vi "Notifier to Command String.vi"(11 "NotifierReff":T1) -> (3 "String":string)   [LabVIEW 2013]
doc: "Takes the MB sail and rudder commands (-1 to 1 for rudder, 0 to 1 for sails) and translates that into a command string for the arbotix board.\n\nEric Schneider, April 2014"
uses:
  Data/TypeDefs/Notifiers.ctl
  Data/TypeDefs/UTM Location.ctl
  Data/TypeDefs/Sail Set Suggestions.ctl
  Data/TypeDefs/Rudder Set Suggestions.ctl
  Data/TypeDefs/OverrideInformation.ctl
  Data/TypeDefs/OverrideMode.ctl
  Data/TypeDefs/MotorSetup.ctl
  Data/TypeDefs/DynamixelSetupInfo.ctl
  Data/TypeDefs/AirmarStatus.ctl
  Data/TypeDefs/HardwareOnline.ctl
  Data/TypeDefs/DynamixelCycleTracker.ctl
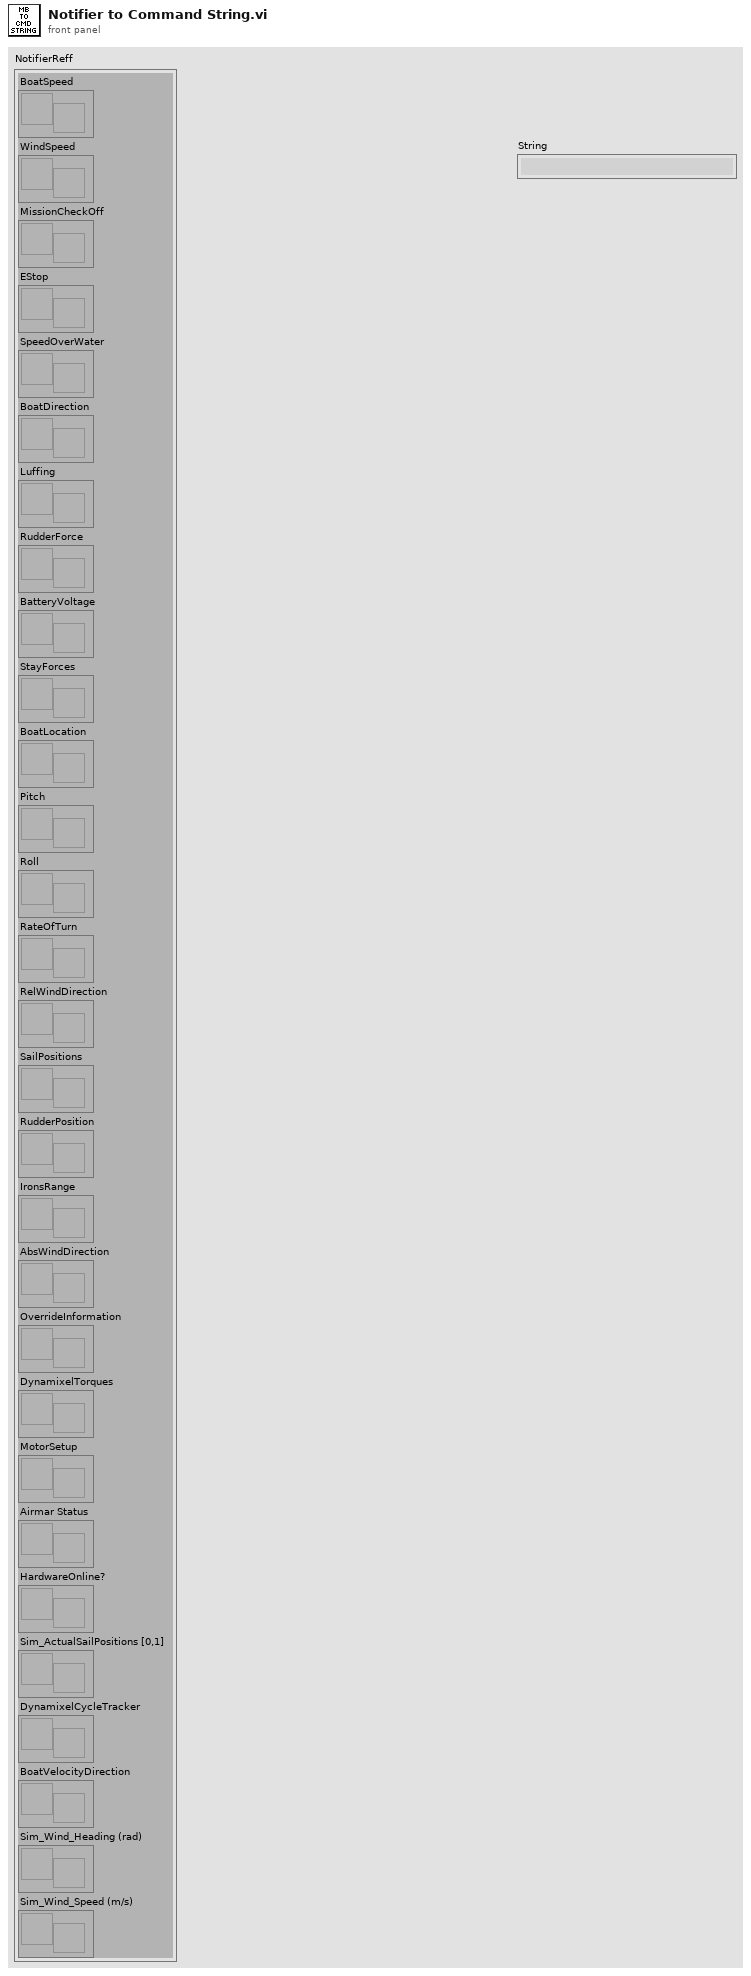
[diagram p1: front panel]
types:
  T1 = typedef "Notifiers.ctl" = cluster{"BoatSpeed":refnum<notifier>, "WindSpeed":refnum<notifier>, "MissionCheckOff":refnum<notifier>, "EStop":refnum<notifier>, "SpeedOverWater":refnum<notifier>, "BoatDirection":refnum<notifier>, "Luffing":refnum<notifier>, "RudderForce":refnum<notifier>, "BatteryVoltage":refnum<notifier>, "StayForces":refnum<notifier>, "BoatLocation":refnum<notifier>, "Pitch":refnum<notifier>, "Roll":refnum<notifier>, "RateOfTurn":refnum<notifier>, "RelWindDirection":refnum<notifier>, "SailPositions":refnum<notifier>, "RudderPosition":refnum<notifier>, "IronsRange":refnum<notifier>, "AbsWindDirection":refnum<notifier>, "OverrideInformation":refnum<notifier>, "DynamixelTorques":refnum<notifier>, "MotorSetup":refnum<notifier>, "Airmar Status":refnum<notifier>, "HardwareOnline?":refnum<notifier>, "Sim_ActualSailPositions [0,1]":refnum<notifier>, "DynamixelCycleTracker":refnum<notifier>, "BoatVelocityDirection":refnum<notifier>, "Sim_Wind_Heading (rad)":refnum<notifier>, "Sim_Wind_Speed (m/s)":refnum<notifier>}
  T2 = typedef "OverrideInformation.ctl" = cluster{"OverrideMode":T3, "SailSetting":T4, "Rudder Setpoint":T5}
  T3 = typedef "OverrideMode.ctl" = enum16{"None", "Rudder", "Sails", "Both"}
  T4 = typedef "Sail Set Suggestions.ctl" = cluster{"MainSailSuggestion":dbl, "JibSailSuggestion":dbl}
  T5 = typedef "Rudder Set Suggestions.ctl" = dbl
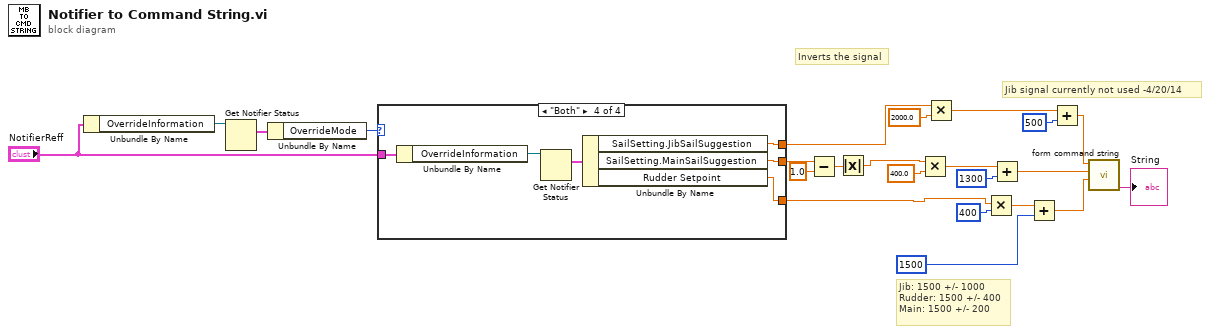
[diagram p0: block diagram]
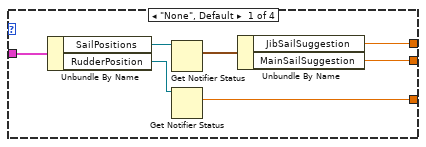
[diagram p2: hidden frame]
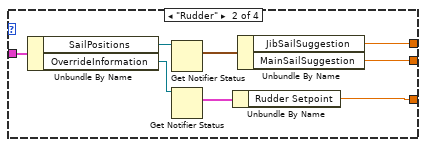
[diagram p3: hidden frame]
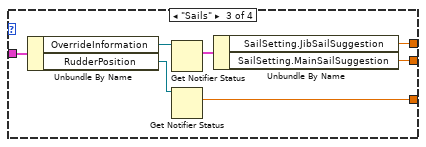
[diagram p4: hidden frame]
diagram:
  # "Jib signal currently not used -4/20/14"
  # "Inverts the signal"
  # "Jib: 1500 +/- 1000\nRudder: 1500 +/- 400\nMain: 1500 +/- 200"
  n1 = Unbundle By Name("NotifierReff") -> ("OverrideInformation"=w8:refnum<notifier>)
  n2 = Get Notifier Status(notifier=w8) -> (current notification=w7:T2)  [unwired: 1 in, 4 out]
  n3 = Unbundle By Name(w7) -> ("OverrideMode"=w6:T3)
  n4 = case shown="\"Both\"" w6 {
    tunnel: "NotifierReff" -> [w28 w38 w45 w51]
    tunnel: [w26 w31 w43 w46] -> w5
    tunnel: [w25 w34 w40 w48] -> w16
    tunnel: [w24 w33 w39 w47] -> w4
    frame "None", Default {
      n5 = Unbundle By Name(w28) -> ("SailPositions"=w30:refnum<notifier>, "RudderPosition"=w29:refnum<notifier>)
      n6 = Get Notifier Status(notifier=w30) -> (current notification=w27:T4)  [unwired: 1 in, 4 out]
      n7 = Get Notifier Status(notifier=w29) -> (current notification=w26:T5)  [unwired: 1 in, 4 out]
      n8 = Unbundle By Name(w27) -> ("JibSailSuggestion"=w25:dbl, "MainSailSuggestion"=w24:dbl)
    }
    frame "Rudder" {
      n9 = Unbundle By Name(w38) -> ("SailPositions"=w37:refnum<notifier>, "OverrideInformation"=w36:refnum<notifier>)
      n10 = Get Notifier Status(notifier=w37) -> (current notification=w35:T4)  [unwired: 1 in, 4 out]
      n11 = Get Notifier Status(notifier=w36) -> (current notification=w32:T2)  [unwired: 1 in, 4 out]
      n12 = Unbundle By Name(w32) -> ("Rudder Setpoint"=w31:T5)
      n13 = Unbundle By Name(w35) -> ("JibSailSuggestion"=w34:dbl, "MainSailSuggestion"=w33:dbl)
    }
    frame "Sails" {
      n14 = Unbundle By Name(w45) -> ("OverrideInformation"=w42:refnum<notifier>, "RudderPosition"=w44:refnum<notifier>)
      n15 = Get Notifier Status(notifier=w42) -> (current notification=w41:T2)  [unwired: 1 in, 4 out]
      n16 = Get Notifier Status(notifier=w44) -> (current notification=w43:T5)  [unwired: 1 in, 4 out]
      n17 = Unbundle By Name(w41) -> ("SailSetting.JibSailSuggestion"=w40:dbl, "SailSetting.MainSailSuggestion"=w39:dbl)
    }
    frame "Both" {
      n18 = Unbundle By Name(w51) -> ("OverrideInformation"=w50:refnum<notifier>)
      n19 = Get Notifier Status(notifier=w50) -> (current notification=w49:T2)  [unwired: 1 in, 4 out]
      n20 = Unbundle By Name(w49) -> ("SailSetting.JibSailSuggestion"=w48:dbl, "SailSetting.MainSailSuggestion"=w47:dbl, "Rudder Setpoint"=w46:T5)
    }
  }
  n21 = Subtract(x=w4, y=1.0) -> (x-y=w2:dbl)
  n22 = Absolute Value(x=w2) -> (abs(x)=w1:dbl)
  n23 = Multiply(x=w1, y=400.0) -> (x*y=w11:dbl)
  n24 = Multiply(x=w16, y=2000.0) -> (x*y=w15:dbl)
  n25 = Multiply(x=w5, y=400) -> (x*y=w20:T5)
  n26 = Add(x=w11, y=1300) -> (x+y=w10:dbl)
  n27 = Add(x=w20, y=1500) -> (x+y=w19:T5)
  n28 = Add(x=w15, y=500) -> (x+y=w14:dbl)
  n29 = call "form command string.vi"("Rudder"=w19, "Main sheet"=w10, "Jib Sheet"=w14) -> ("String"=→"String":string)  [unwired: 5 in, 3 out]
